vi "Initialize.vi"(6 "firmware revision":string, 7 "Serial Configuration":T1={"Baud Rate"=9600, "Parity"=0, "Data Bits"=8, "Stop Bits"=10, "Flow Control"=0} {"Flow Control" items=["None", "XON/XOFF", "RTS/CTS", "XON/XOFF & RTS/CTS", "DTR/DSR", "XON/XOFF & DTR/DSR"]; "Stop Bits" items=["1.0"=10, "1.5"=15, "2.0"=20]; "Data Bits" items=["7"=7, "8"=8]; "Parity" items=["None", "Odd", "Even", "Mark", "Space"]; "Baud Rate" items=["300"=300, "600"=600, "1200"=1200, "2400"=2400, "4800"=4800, "9600"=9600, "19200"=19200, "38400"=38400, "57600"=57600, "115200"=115200]}, 8 "error in (no error)":errorcluster, 9 "Reset (True)":bool=TRUE, 10 "ID Query (True)":bool=TRUE, 11 "VISA resource name":refnum<visa-resource-name>) -> (0 "error out":errorcluster, 2 "firmware revision":string, 3 "VISA resource name out":refnum<visa-resource-name>)   [LabVIEW 2021, in "Andeen-Hagerling 2700A.lvlib"]
doc: "Establishes communication with the instrument and optionally performs an instrument identification query and/or an instrument reset. It also places the instrument in a default state needed for other instrument driver operations. Therefore, call this VI before calling other instrument driver VIs for this instrument. Generally, you need to call the Initialize VI only once at the beginning of an application."
uses:
  Andeen-Hagerling 2700A.lvlib
panel:
  # "(c) 2006 ANDEEN-HAGERLING, INC.  ALL RIGHTS RESERVED."
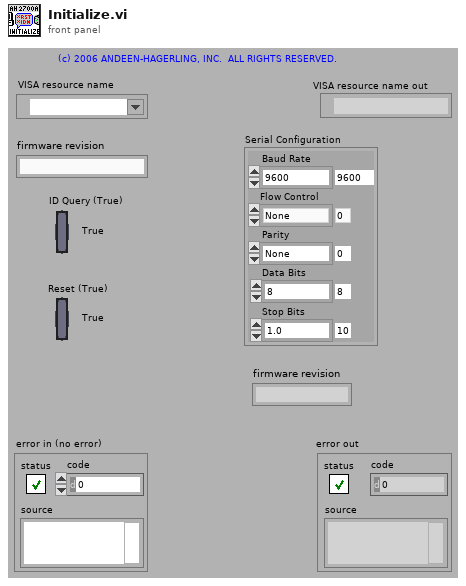
[diagram p1: front panel]
types:
  T1 = cluster{"Baud Rate":u32, "Parity":u16, "Data Bits":u16, "Stop Bits":u16, "Flow Control":u16}
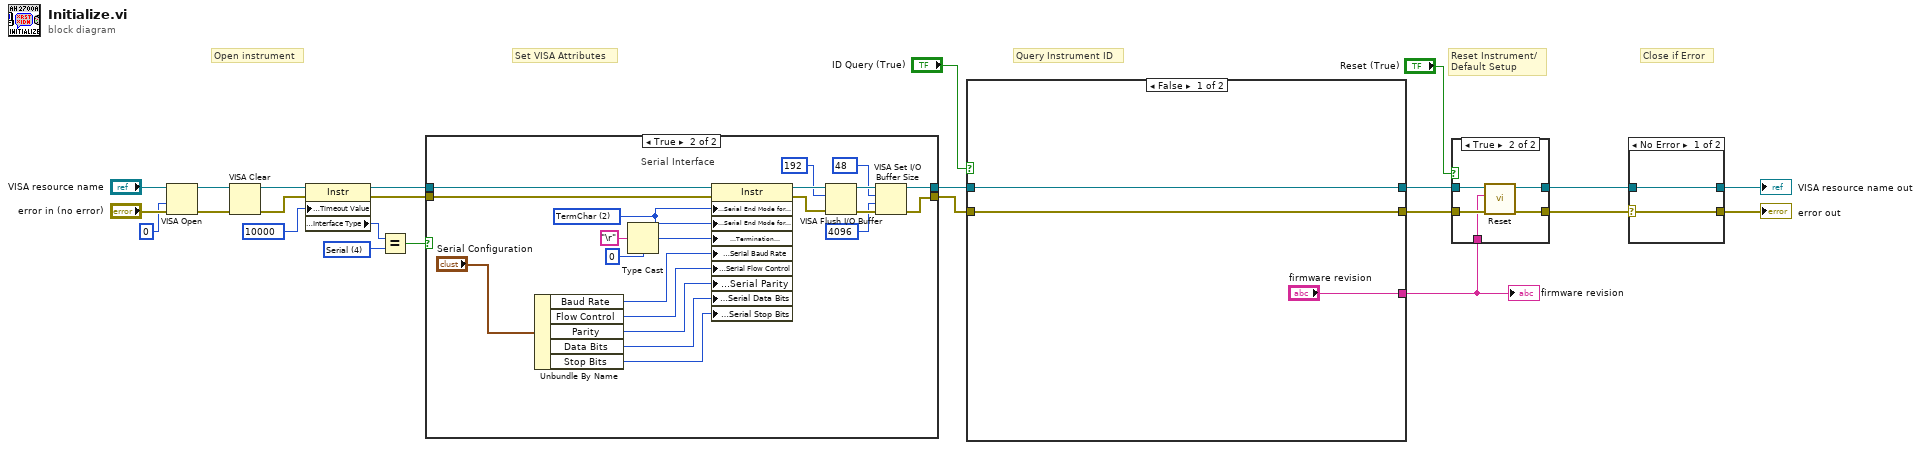
[diagram p0: block diagram]
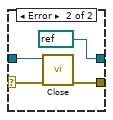
[diagram p3: hidden frame]
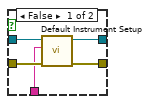
[diagram p4: hidden frame]
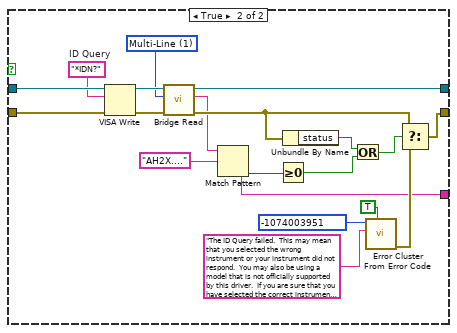
[diagram p5: hidden frame]
diagram:
  w11 = u16 4 items=["GPIB"=1, "VXI"=2, "GPIB-VXI"=3, "Serial"=4, "PXI"=5, "TCPIP"=6, "USB"=7] ("Interface Information:Interface Type")
  # "Set VISA Attributes"
  # "Close if Error"
  # "Query Instrument ID"
  # "Reset Instrument/\nDefault Setup"
  # "Open instrument"
  n1 = VISA Open(access mode=u32 0, error in (no error)="error in (no error)", VISA resource name="VISA resource name") -> (VISA resource name=w9:refnum<visa-resource-name>, error out=w8:errorcluster)  [unwired: 2 in]
  n2 = VISA Clear(VISA resource name=w9, error in (no error)=w8) -> (VISA resource name out=w7:refnum<visa-resource-name>, error out=w6:errorcluster)
  n3 = property class="Instr"(reference=w7, error in=w6, "General Settings:Timeout Value"=u32 10000) -> (reference out=w14:refnum<visa-resource-name>, error out=w13:errorcluster, "Interface Information:Interface Type"=w18:u16)
  n4 = Equal?(x=w18, y=w11) -> (x = y?=w12:bool)
  n5 = case shown="True" w12 {
    tunnel: [w25 w44] -> w16
    tunnel: [w26 w41] -> w15
    tunnel: w14 -> [w25 w46]
    tunnel: w13 -> [w26 w47]
    frame False {
      # "EDIT: Remove interfaces not\nsupported by your instrument."
      # "GPIB, TCP/IP, and USB Interface"
    }
    frame True {
      w34 = u16 2 items=["None", "LastBit", "TermChar"] ("Serial Settings:Serial End Mode for Reads")
      # "Serial Interface"
      n6 = Unbundle By Name("Serial Configuration") -> ("Baud Rate"=w32:u32, "Flow Control"=w28:u16, "Parity"=w30:u16, "Data Bits"=w31:u16, "Stop Bits"=w27:u16)
      n7 = Type Cast(type=u8 0, x="\r") -> (*(type *) &x=w33:u8)
      n8 = property class="Instr"(reference=w46, error in=w47, "Serial Settings:Serial End Mode for Reads"=w34, "Serial Settings:Serial End Mode for Writes"=w34, "Message Based Settings:Termination Character"=w33, "Serial Settings:Serial Baud Rate"=w32, "Serial Settings:Serial Flow Control"=w28, "Serial Settings:Serial Parity"=w30, "Serial Settings:Serial Data Bits"=w31, "Serial Settings:Serial Stop Bits"=w27) -> (reference out=w40:refnum<visa-resource-name>, error out=w43:errorcluster)
      n9 = VISA Flush I/O Buffer(VISA resource name=w40, mask (16)=u16 192, error in (no error)=w43) -> (VISA resource name out=w45:refnum<visa-resource-name>, error out=w42:errorcluster)
      n10 = VISA Set I/O Buffer Size(VISA resource name=w45, mask (16)=u16 48, size (4096)=u32 4096 ("size (0)"), error in (no error)=w42) -> (VISA resource name out=w44:refnum<visa-resource-name>, error out=w41:errorcluster)
    }
  }
  n11 = case shown="False" "ID Query (True)" {
    tunnel: [w49 w70] -> w23
    tunnel: [w50 w54] -> w24
    tunnel: w16 -> [w50 w68]
    tunnel: w15 -> [w49 w69]
    tunnel: ["firmware revision" w57] -> w1
    frame False {
    }
    frame True {
      w51 = u16 1 items=["Single Line", "Multi-Line"] ("Multiline")
      w67 = "*IDN?"  # ID Query
      n12 = VISA Write(VISA resource name=w68, write buffer=w67, error in (no error)=w69) -> (VISA resource name out=w56:refnum<visa-resource-name>, error out=w55:errorcluster)  [unwired: 1 out]
      n13 = call "Bridge Read.vi"("error in (no error)"=w55, "multiline"=w51, "VISA resource name"=w56) -> ("error out"=w53:errorcluster, "read buffer"=w52:string, "VISA resource name out"=w54:refnum<visa-resource-name>)  [unwired: 6 in]
      n14 = Match Pattern(string=w52, regular expression="AH2X....") -> (match substring=w57:string, offset past match=w62:i32)  [unwired: 1 in, 2 out]
      n15 = Greater Or Equal To 0?(x=w62) -> (x >= 0?=w60:bool)
      n16 = Unbundle By Name(w53) -> ("status"=w61:bool)
      n17 = Or(x=w61, y=w60) -> (x .or. y?=w59:bool)
      n18 = call <vilib>:"Error Cluster From Error Code.vi"("show call chain? (False)"=TRUE, "error message (\"\")"="The ID Query failed.  This may mean that you selected the wrong instrument or your instrument did not respond.  You may also be using a model that is not officially supported by this driver.  If you are sure that you have selected the correct instrument and it is responding, try disabling the ID Query." ("Source (VI Name)"), "error code (0)"=-1074003951 ("Code")) -> ("error out"=w66:errorcluster)  [unwired: 6 in]
      n19 = Select(t=w53, s=w59, f=w66) -> (s? t:f=w70:errorcluster)
    }
  }
  "firmware revision" <- w1
  n20 = case shown="True" "Reset (True)" {
    tunnel: w23 -> [w74 w77]
    tunnel: [w73 w80] -> w2
    tunnel: w24 -> [w75 w78]
    tunnel: [w72 w79] -> w3
    tunnel: w1 -> [w71 w76]
    frame False {
      n21 = call "Default Instrument Setup.vi"("error in (no error)"=w74, "firmware revision"=w71, "VISA resource name"=w75) -> ("error out"=w73:errorcluster, "VISA resource name out"=w72:refnum<visa-resource-name>)  [unwired: 7 in]
    }
    frame True {
      n22 = call "Reset.vi"("error in (no error)"=w77, "firmware revision"=w76, "VISA resource name"=w78) -> ("error out"=w80:errorcluster, "VISA resource name out"=w79:refnum<visa-resource-name>)  [unwired: 7 in]
    }
  }
  n23 = case shown="No Error" w2 {
    selector: w2 -> [w82 w84]
    tunnel: w3 -> [w81 w85]
    tunnel: [w81 refnum<visa-resource-name> refnum ("VISA resource name out")] -> w5
    tunnel: [w82 w86] -> w4
    frame No Error {
    }
    frame Error {
      n24 = call "Close.vi"("error in (no error)"=w84, "VISA resource name"=w85) -> ("error out"=w86:errorcluster)  [unwired: 9 in]
    }
  }
  "VISA resource name out" <- w5
  "error out" <- w4
